vi "RollValidate.vi"() -> ()   [LabVIEW 2016]
uses:
  <vilib>/myRIO/Instrument Drivers/Onboard IO/UART/typedef/VISA Configuration.ctl
  <vilib>/myRIO/Instrument Drivers/Onboard IO/DIO/typedefs/DIO Reference.ctl
  <vilib>/myRIO/Common/Instrument Driver Framework/Utilities/typedefs/myRIO Generic Hardware Reference.ctl
  <vilib>/myRIO/Common/Instrument Driver Framework/Utilities/typedefs/Hardware Version Enum.ctl
  <vilib>/myRIO/Common/Instrument Driver Framework/Utilities/typedefs/myRIO v1.0 Reference.ctl
  <vilib>/myRIO/Common/Instrument Driver Framework/Utilities/typedefs/Generic FPGA Reference.ctl
  <vilib>/myRIO/Common/Instrument Driver Framework/myRIO v1.0/DIO/typedefs/DIO Channels List.ctl
  <vilib>/myRIO/Common/Instrument Driver Framework/myRIO v1.0/DIO/typedefs/DIO Channels Enum.ctl
  <vilib>/userdefined/High Color/nirio_resource_hc.ctl
  <vilib>/myRIO/Common/Instrument Driver Framework/Utilities/vis/Is FPGA Ref Available.vi
  <vilib>/myRIO/Common/Instrument Driver Framework/roboRIO v1.0/DIO/vis/roboRIO v1.0 Open DIO.vi
  <vilib>/myRIO/Instrument Drivers/Onboard IO/DIO/vis/Write.vi
  <vilib>/myRIO/Common/Instrument Driver Framework/Utilities/vis/Validate Channels.vi
  <vilib>/myRIO/Common/Instrument Driver Framework/roboRIO v1.0/DIO/vis/roboRIO v1.0 Reserve DIO.vi
  <vilib>/myRIO/Common/Instrument Driver Framework/roboRIO v1.0/DIO/vis/roboRIO v1.0 Build MUX Configuration DIO.vi
  <vilib>/myRIO/Common/Instrument Driver Framework/roboRIO v1.0/Resource Manager/vis/roboRIO v1.0 Reserve Channel List.vi
  <vilib>/myRIO/Common/Instrument Driver Framework/roboRIO v1.0/Resource Manager/vis/roboRIO v1.0 Create Configuration List.vi
  <vilib>/myRIO/Common/Instrument Driver Framework/roboRIO v1.0/Resource Manager/vis/roboRIO v1.0 Reserve Channel.vi
  <vilib>/myRIO/Common/Instrument Driver Framework/roboRIO v1.0/Resource Manager/vis/roboRIO v1.0 Unreserve Channel.vi
  <vilib>/myRIO/Common/Instrument Driver Framework/roboRIO v1.0/Resource Manager/vis/roboRIO v1.0 Build Mutex Name.vi
  <vilib>/Instr/_visa.llb/VISA Configure Serial Port (Instr).vi
  <vilib>/Utility/VariantDataType/GetNumericInfo.vi
  <vilib>/Utility/error.llb/Error Cluster From Error Code.vi
  <vilib>/myRIO/Common/Instrument Driver Framework/roboRIO v1.0/roboRIO v1.0 Open.vi
  <vilib>/myRIO/Common/Instrument Driver Framework/Utilities/vis/IO Manager.vi
  <vilib>/myRIO/Common/Instrument Driver Framework/Utilities/vis/Configuration Manager.vi
  <vilib>/myRIO/Common/Instrument Driver Framework/roboRIO v1.0/Resource Manager/vis/roboRIO v1.0 Configure IO.vi
  <vilib>/myRIO/Common/Instrument Driver Framework/myRIO v1.0/myRIO v1.0 Close.vi
  <vilib>/myRIO/Common/Instrument Driver Framework/roboRIO v1.0/DIO/vis/roboRIO v1.0 Write DIO.vi
  <vilib>/myRIO/Express VI/Onboard IO/UART/UART Express VI.xnode
  <vilib>/myRIO/Express VI/Onboard IO/DO/DO Express VI.xnode
  <vilib>/myRIO/Instrument Drivers/Onboard IO/DIO/vis/myRIO DIO Open.xnode
  <vilib>/myRIO/Instrument Drivers/Onboard IO/UART/UART.lvlib
  <vilib>/myRIO/Instrument Drivers/Onboard IO/DIO/DIO.lvlib
panel:
  out "Empty buffer":string
  in  "Stop":bool
  in  "Power on IMU":bool
  out "Roll angle":dbl(knob) scale=-90.0..90.0
  out "Lean Angle":dbl
  out "Characters Read":string
  out "Time":dbl format="%.2f"
  in  "SteeringAngle":dbl
  in  "v":dbl
  out "Bias":T1
  out "error out":errorcluster
  in  "Start":bool
  out "Roll":dbl
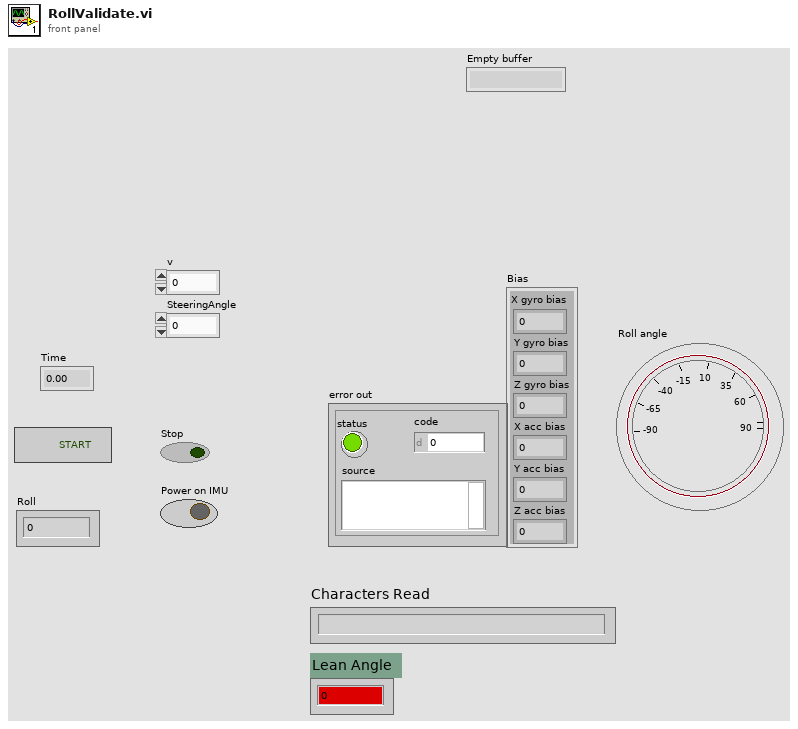
[diagram p1: front panel]
types:
  T1 = cluster{"X gyro bias":dbl, "Y gyro bias":dbl, "Z gyro bias":dbl, "X acc bias":dbl, "Y acc bias":dbl, "Z acc bias":dbl}
  T2 = typedef "UART.lvlib/VISA Configuration.ctl" = cluster{"baud rate (9600)":u32, "data bits (8)":u16, "parity (0:none)":enum16{"None", "Odd", "Even", "Mark", "Space"}, "stop bits (10: 1 bit)":u16, "flow control (0:none)":u16, "termination char\n(0xA = '\\n' = LF) ":u8, "Enable Termination\nChar (T)":bool, "timeout (10sec)":u32}
  T3 = enum16{"open", "open or create", "create or replace", "create", "open (read-only)"}
  T4 = cluster{"FilteredGyroX":dbl, "FilteredGyroY":dbl}
  T5 = typedef "DIO.lvlib/DIO Reference.ctl" = cluster{"myRIO Reference":T6, "DIO Channels List":T10}
  T6 = typedef "myRIO Generic Hardware Reference.ctl" = cluster{"myRIO Model":T7, "myRIO Hardware Reference":T8}
  T7 = typedef "Hardware Version Enum.ctl" = enum16{"Unknown", "myRIO-1900", "myRIO-1950", "roboRIO", "NI ELVIS RIO CM"}
  T8 = typedef "myRIO v1.0 Reference.ctl" = cluster{"Generic FPGA Reference":T9, "Allow multiple opens":bool}
  T9 = typedef "Generic FPGA Reference.ctl" = refnum<k20>
  T10 = typedef "DIO Channels List.ctl" = T11[]
  T11 = typedef "DIO Channels Enum.ctl" = enum16{"Not Connected", "C/DIO0", "C/DIO1", "C/DIO2", "C/DIO3", "C/DIO4", "C/DIO5", "C/DIO6", "C/DIO7", "A/DIO0", "A/DIO1", "A/DIO2", "A/DIO3", "A/DIO4", "A/DIO5", "A/DIO6", "A/DIO7", "A/DIO8", "A/DIO9", "A/DIO10", "A/DIO11", "A/DIO12", "A/DIO13", "A/DIO14", "A/DIO15", "B/DIO0", "B/DIO1", "B/DIO2", "B/DIO3", "B/DIO4", "B/DIO5", "B/DIO6", "B/DIO7", "B/DIO8", "B/DIO9", "B/DIO10", "B/DIO11", "B/DIO12", "B/DIO13", "B/DIO14", "B/DIO15", "LED0", "LED1", "LED2", "LED3", "Button0", "DIO/DIO0", "DIO/DIO1", "DIO/DIO2", "DIO/DIO3", "DIO/DIO4", "DIO/DIO5", "DIO/DIO6", "DIO/DIO7", "DIO/DIO8", "DIO/DIO9", "SPI/CS0", "SPI/CS1", "SPI/CS2", "SPI/CS3", "LED RADIO (Green)", "LED RADIO (Red)", "LED COMM (Green)", "LED COMM (Red)", "LED MODE (Green)", "LED MODE (Red)"}
  T12 = typedef "nirio_resource_hc.ctl" = tag
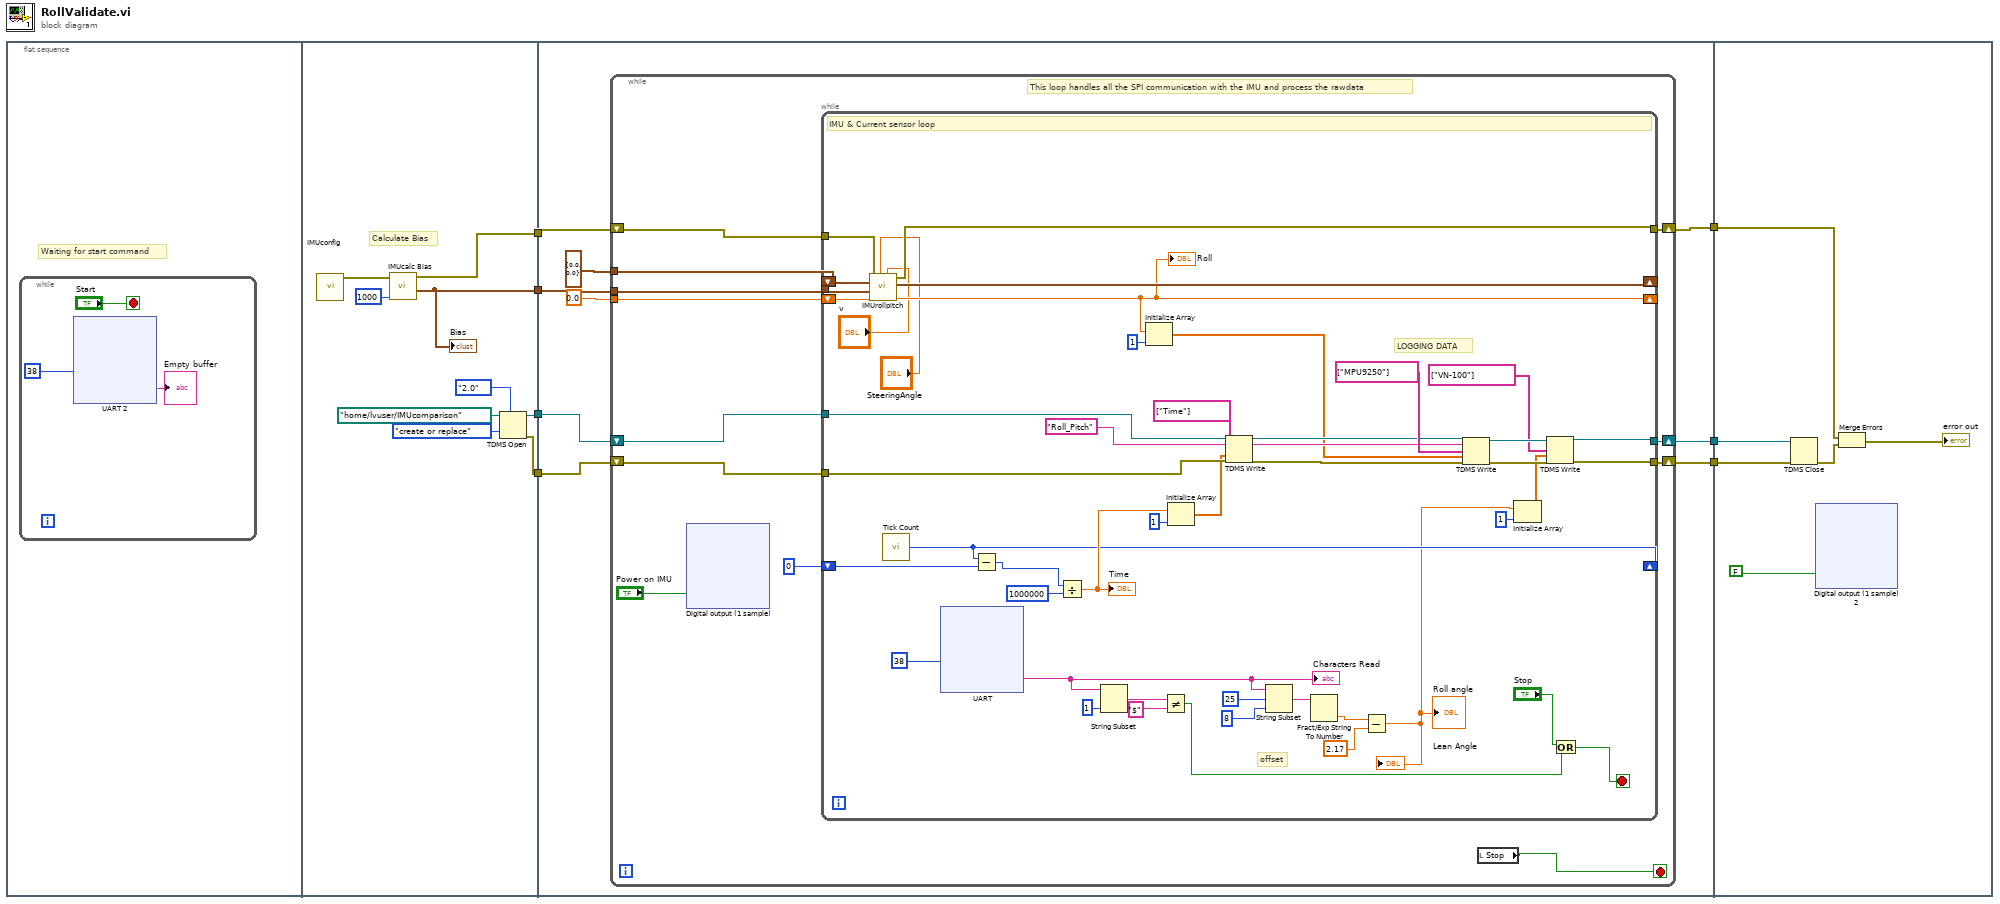
[diagram p0: block diagram]
diagram:
  n1 = flat-sequence {
    tunnel: [w35] -> w7
    tunnel: [w34] -> w6
    tunnel: [w32] -> w5
    tunnel: [w31] -> w4
    tunnel: w7 -> [w43]
    tunnel: w6 -> [w42]
    tunnel: w5 -> [w41]
    tunnel: w4 -> [w40]
    tunnel: [w39] -> w3
    tunnel: [w38] -> w2
    tunnel: [w37] -> w1
    tunnel: w3 -> [w159]
    tunnel: w2 -> [w158]
    tunnel: w1 -> [w157]
    frame #0 {
      # "Waiting for start command"
      n2 = while {
        stop <- "Start" stop-if-true
        n3 = xnode "UART 2"("Character Count"=u32 38) -> ("Characters Read"=→"Empty buffer":string)  [unwired: 1 in, 1 out]
      }
    }
    frame #1 {
      # "Calculate Bias"
      n4 = call "IMUconfig.vi"() -> ("error out"=w27:errorcluster)  [unwired: 11 in]
      n5 = call "IMUcalc Bias.vi"("Number of loops"=1000, "error in (no error)"=w27) -> ("Bias"=w35:T1, "error out"=w34:errorcluster)  [unwired: 7 in]
      "Bias" <- w35
      n6 = TDMS Open(7:enum16{"1.0", "2.0"}."2.0" ("file format version (2.0)"), 10:T3."create or replace" ("operation (0:open)"), 11:path "/home/lvuser/IMUcomparison" ("file path")) -> (0:w31:errorcluster, 3:w32:refnum<k34>)  [unwired: 4 in]
    }
    frame #2 {
      n7 = while {
        tunnel: 0.0 ("xAngle in") -> [w56]
        tunnel: w43 -> [w55]
        tunnel: T4 {"FilteredGyroX"=0.0, "FilteredGyroY"=0.0} ("FilteredGyro") -> [w48]
        shift-right: [w49] -> w37
        shift-left: w42 -> [w54]
        shift-right: [w51] -> w39
        shift-left: w41 -> [w53]
        shift-right: [w50] -> w38
        shift-left: w40 -> [w52]
        stop <- w45 stop-if-true
        # "This loop handles all the SPI communication with the IMU and process the rawdata"
        n8 = xnode "Digital output (1 sample)"("DIO/DIO3 (Pin 3)"="Power on IMU") -> ()  [unwired: 1 in, 1 out]
        n9 = while {
          tunnel: w55 -> [w127]
          tunnel: w54 -> [w138]
          shift-right: [w122] -> _
          shift-left: w56 -> [w126]
          tunnel: [w137] -> w49
          tunnel: w53 -> [w132]
          tunnel: w52 -> [w131]
          tunnel: [w105] -> w51
          tunnel: [w106] -> w50
          shift-right: [w125] -> _
          shift-left: w48 -> [w123]
          shift-right: [w95] -> _
          shift-left: u32 0 ("y") -> [w119]
          stop <- w99 stop-if-true
          # "offset"
          # "LOGGING DATA"
          # "IMU & Current sensor loop"
          n10 = call "IMUrollpitch.vi"("v(m/s)"="v", "SteeringAngle(rad/s)"="SteeringAngle", "PrevRoll(deg)"=w126, "Bias"=w127, "PrevFilteredGyro(deg)"=w123, "error in (no error)"=w138) -> ("Roll(deg)"=w122:dbl, "FilteredGyro(deg)"=w125:T4, "error out"=w137:errorcluster)  [unwired: 3 in]
          "Roll" <- w122
          n11 = call "Tick Count"() -> ("Tick Count(uSec)"=w95:u32)
          n12 = xnode "UART"("Character Count"=u32 38) -> ("Characters Read"=w113:string)  [unwired: 1 in, 1 out]
          "Characters Read" <- w113
          n13 = Subtract(x=w95, y=w119) -> (x-y=w98:u32)
          n14 = Divide(x=w98, y=u32 1000000) -> (x/y=w96:dbl)
          "Time" <- w96
          n15 = String Subset(string=w113, length (rest)=1 ("length (rest)")) -> (substring=w111:string)  [unwired: 1 in]
          n16 = Initialize Array(w122, 1 ("dimension size")) -> (w124:dbl[])
          n17 = Not Equal?(x=w111, y="$") -> (x != y?=w100:bool)
          n18 = Initialize Array(w96, 1 ("dimension size")) -> (w117:dbl[])
          n19 = TDMS Write(0:w132, 5:"Roll_Pitch" ("group name in (Untitled)"), 7:string[] ["Time"] ("channel name(s) in (Untitled)"), 9:w117, 11:w131) -> (4:w128:refnum<k34>, 6:w130:string, 15:w129:errorcluster)  [unwired: 1 in, 1 out]
          n20 = String Subset(string=w113, offset (0)=25, length (rest)=8 ("length (rest)")) -> (substring=w109:string)
          n21 = Fract/Exp String To Number(string=w109) -> (number=w94:dbl)  [unwired: 3 in, 1 out]
          n22 = Subtract(x=w94, y=2.17) -> (x-y=w93:dbl)
          "Lean Angle" <- w93
          "Roll angle" <- w93
          n23 = TDMS Write(0:w128, 5:w130, 7:string[] ["MPU9250"] ("channel name(s) in (Untitled)"), 9:w124, 11:w129) -> (4:w108:refnum<k34>, 15:w107:errorcluster)  [unwired: 1 in, 2 out]
          n24 = Initialize Array(w93, 1 ("dimension size")) -> (w104:dbl[])
          n25 = TDMS Write(0:w108, 7:string[] ["VN-100"] ("channel name(s) in (Untitled)"), 9:w104, 11:w107) -> (4:w105:refnum<k34>, 15:w106:errorcluster)  [unwired: 2 in, 2 out]
          n26 = Or(x="Stop", y=w100) -> (x .or. y?=w99:bool)
        }
        n27 = local read "Stop"() -> (w45:bool)
      }
    }
    frame #3 {
      n28 = TDMS Close(8:w158, 11:w159) -> (0:w160:errorcluster)  [unwired: 1 out]
      n29 = xnode "Digital output (1 sample) 2"("DIO/DIO3 (Pin 3)"=FALSE) -> ()  [unwired: 1 in, 1 out]
      n30 = Merge Errors(w157, w160) -> (→"error out":errorcluster)
    }
  }
